vi "Image Marked Areas.vi"(7 "Calling VI Ref":refnum<vi>) -> ()   [LabVIEW 2020]
uses:
  <vilib>/Utility/miscctls.llb/LVPointTypeDef.ctl
  IMA Type Defs/IMA Actions.ctl
  Orca Flash Capture Manager/Orca Flash Capture Manager Controls/Orca Flash Capture Notifier Type.ctl
  Orca Flash Capture Manager/Orca Flash Capture Manager Controls/Orca Flash Capture Actions.ctl
  Orca Flash Capture Manager/Orca Flash Capture Manager Controls/Orca Flash Capture Switch Line Scan Modes.ctl
  Hardware Configuration/Hardware Configuration Controls/Device Function.ctl
  Hardware Configuration/Hardware Configuration Controls/Device Type.ctl
  IMA Type Defs/IMA Marked Positions.ctl
  Wide Field Drift Correction/WFDC Controls/WFDC Notifier Element.ctl
  Wide Field Drift Correction/WFDC Controls/WFDC Actions.ctl
  <vilib>/vision/Image Controls.llb/IMAQ Image.ctl
  Wide Field Drift Correction/WFDC Controls/WFDC External Sync.ctl
  Wide Field Drift Correction/WFDC Controls/WFDC Cycle Pause.ctl
  Wide Field Drift Correction/WFDC Controls/WFDC Status.ctl
  Device Library/Stages/Stages Controls/Stage Actions.ctl
  <vilib>/Utility/error.llb/whitespace.ctl
  8d6d82c7-2c11-4586-8521-e073de89416a.vi
  Device Library/Microscopes/Polymorphic Microscope Messenger/Set Obj Z Pos.vi
  Device Library/Microscopes/Polymorphic Microscope Messenger/Get Obj Z Pos.vi
panel:
  in  "Acquisition Control":enum32{"Capture", "Capture All", "Abort"}(radio)
  in  "Skip":bool
  in  "Clear All":bool
  in  "Clear Selected":bool
  in  "Mark Point":bool
  in  "Marked Positions":i32(listbox)
  in  "Quit":bool
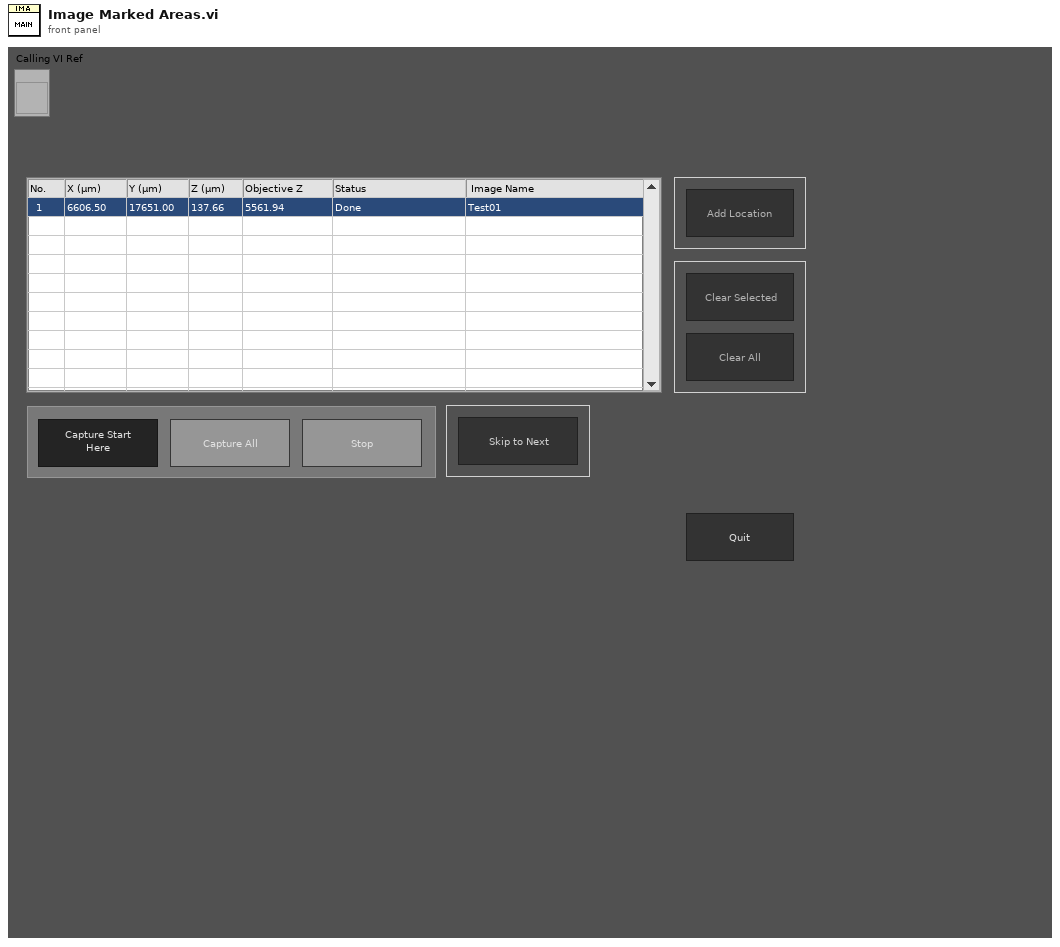
[diagram p1: front panel]
types:
  T1 = typedef "Orca Flash Capture Notifier Type.ctl" = cluster{"Actions":T2, "Running?":bool, "Preview Exposure (s)":dbl, "Capture Exposure (s)":dbl, "Cycles":u16, "Frames":u32, "No. of Z Steps":u16, "Z Step Size (µm)":dbl, "Base Path":path, "Init Z Position (µm)":dbl, "Lasers Lines":string[], "Save Path":path, "Line Scan?":bool, "Line Scan Mode":T3, "Collect Metadata?":bool, "channelCode":u8, "setupName":string, "Presaved Metadata":path}
  T2 = typedef "Orca Flash Capture Actions.ctl" = enum16{"Idle", "Live Preview", "Capture", "Check File Name", "Laser On", "Laser Off", "Open Shutters", "Close Shutters", "Set Exposure Time", "Start Acquisition", "Update SubFolder", "Write Metadata", "Setup", "Camera", "Switch", "Step", "Cycle", "External Cycle Sync", "Abort", "Quit"}
  T3 = typedef "Orca Flash Capture Switch Line Scan Modes.ctl" = enum32{"Automatic", "Use Presets", "Manual"}
  T4 = typedef "IMA Actions.ctl" = enum16{"Add Position", "Update Saved", "Remove Position", "Capture All", "Capture Here", "Move to Position", "Update Name", "Capture", "Switch", "Clear All", "Abort", "Exit Loop", "Quit"}
  T5 = enum16{"Always On", "Always Off", "Off While Running"}
  T6 = typedef "LVPointTypeDef.ctl" = cluster{"Horizontal":i16, "Vertical":i16}
  T7 = enum8{"Enabled", "Disabled", "Disabled and Grayed Out"}
  T8 = typedef "Device Function.ctl" = enum16{"Primary", "Secondary", "Overview", "Wide Field Drift Correction", "642 nm Excitation", "560 nm Excitation", "940 nm Excitation", "546 nm Excitation", "488 nm Excitation", "405 nm Excitation", "Objective Drift Correction", "4Pi Objective Lock", "Objective XY", "Objective Z", "Sample XY", "Sample Coarse Z", "Sample Z", "4Pi Lower", "4Pi Upper", "Mojo", "Adj Cavity", "Line Scanning", "Alert"}
  T9 = typedef "Device Type.ctl" = enum16{"AOTF", "Camera", "Deformable Mirror", "Laser", "Microscope Base", "Shutter", "Stage", "Waveform", "FPGA", "Email", "Filter Wheel", "Spinning Disk"}
  T10 = typedef "WFDC External Sync.ctl" = cluster{"Cycle Sync":T11, "Z Offset":dbl, "WFDC Status":T12}
  T11 = typedef "WFDC Cycle Pause.ctl" = enum16{"Pause Requested", "Paused", "Resume Requested", "Resumed"}
  T12 = typedef "WFDC Status.ctl" = enum16{"Idle", "Busy", "DC Active", "Error", "Canceled"}
  T13 = typedef "WFDC Notifier Element.ctl" = cluster{"WFDC Actions":T14, "Initial XYZ Positions":dbl[], "Ref Images":T15[], "Calibration (slope, inter)":dbl[], "Base Path":path, "Latest Scan Path":path, "Error":errorcluster, "XYZ Drift":dbl[]}
  T14 = typedef "WFDC Actions.ctl" = enum16{"Error Check", "Remote Start", "Move to Pos", "Pre Start Get Drift", "Pre Start Check Drift", "Pre Start Z Drift", "Pre Start XY Drift", "Pre Start ReFocus", "Setup New DC", "Setup Camera", "Get Ref Images", "Calc Calibration", "Switch Tabs", "Get Drift", "Z Drift", "XY Drift", "Start Cycle", "Stop DC", "Abort Remote", "Exit Loop", "Set Error", "Generate Calibration", "Quit"}
  T15 = typedef "IMAQ Image.ctl" = refnum<image>
  T16 = typedef "IMA Marked Positions.ctl" = cluster{"XYZ Positions":string[][], "File Paths":string[]}
  T17 = enum32{"Invalid", "Standard", "Closed", "Hidden", "Minimized", "Maximized"}
  T18 = typedef "Stage Actions.ctl" = enum16{"Get Position", "MVR", "MOVE", "HALT", "ONTARGET", "ERROR", "REFERENCE", "INIT", "VELOCITY", "STATUS", "EXIT", "HOME", "ZEROPOS", "NANOPOS", "ANALOG", "QUIT"}
  T19 = typedef "whitespace.ctl" = u16
  T20 = typedef "LVRectTypeDef.ctl" = cluster{"Left":i16, "Top":i16, "Right":i16, "Bottom":i16}
  T21 = typedef "LVBoundsTypeDef.ctl" = cluster{"Width":u32, "Height":u32}
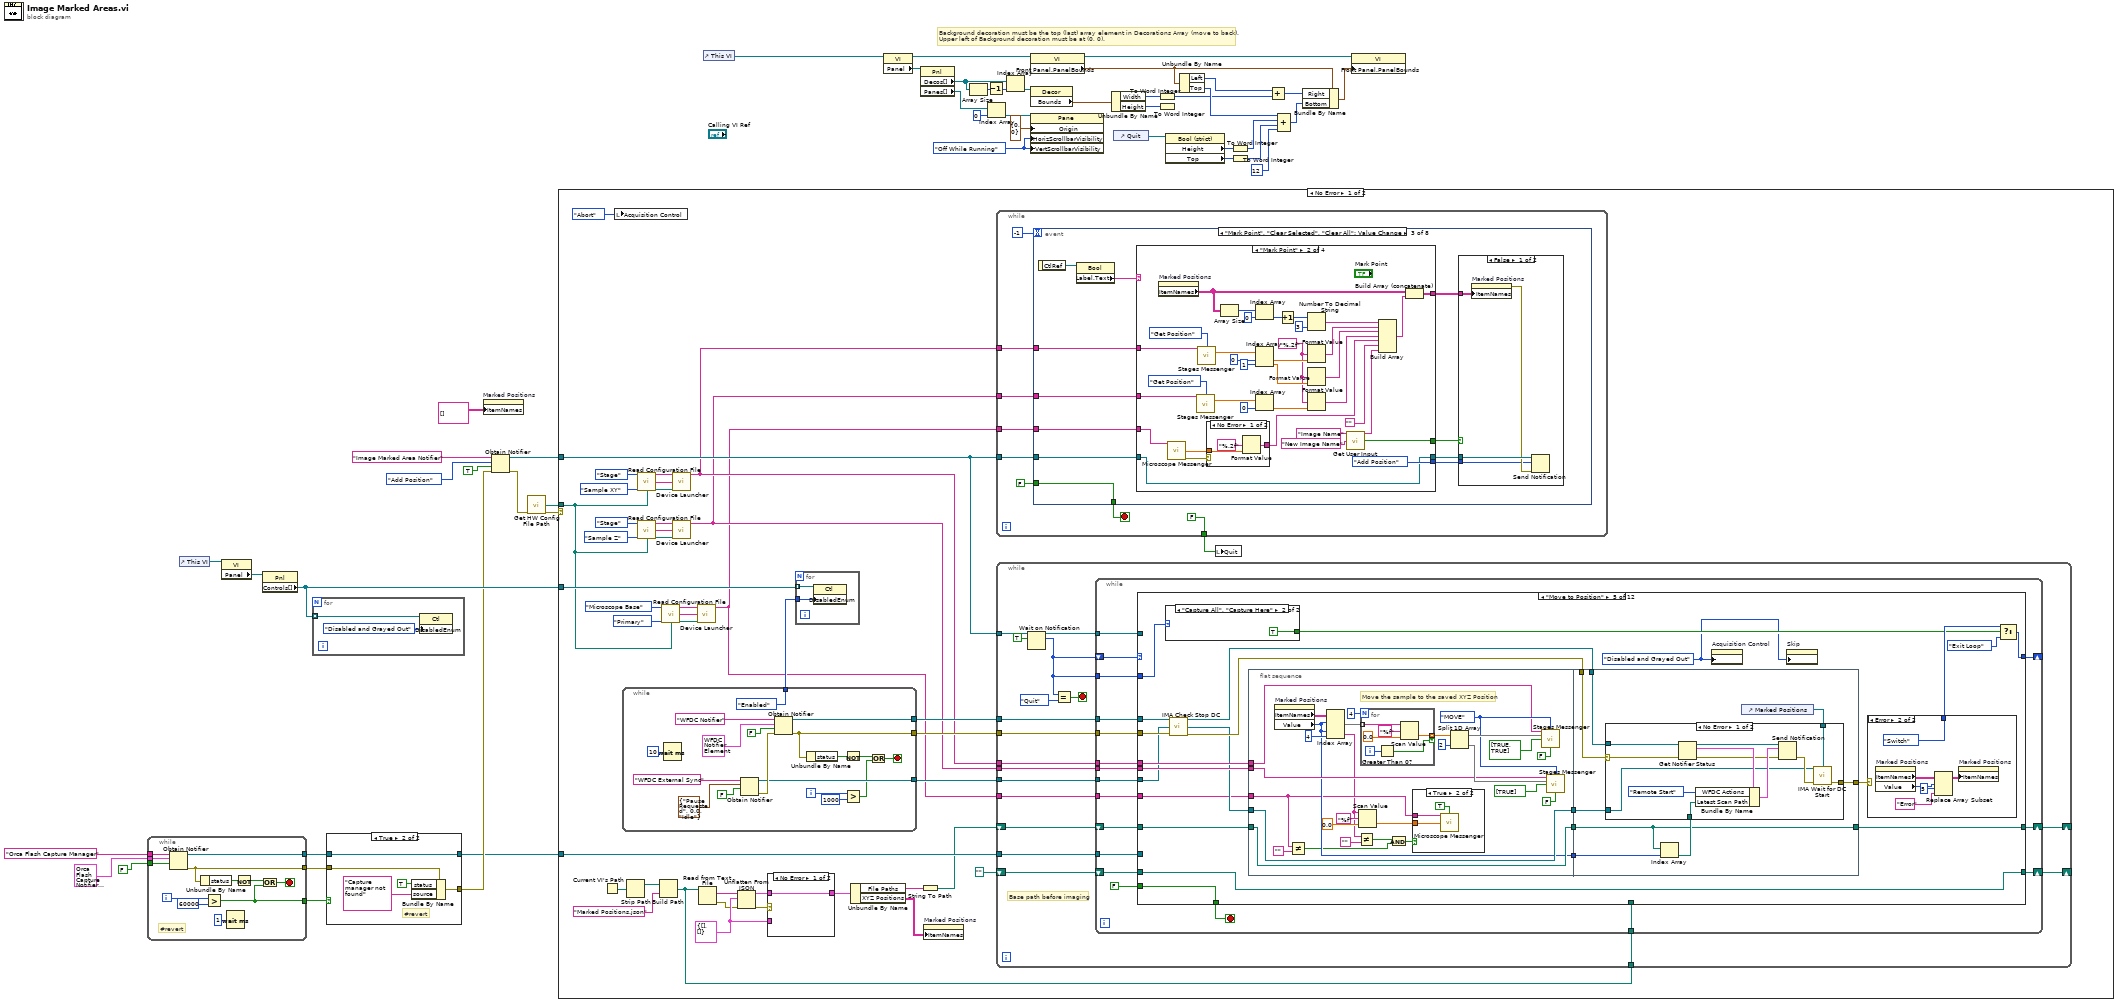
[diagram p0: block diagram]
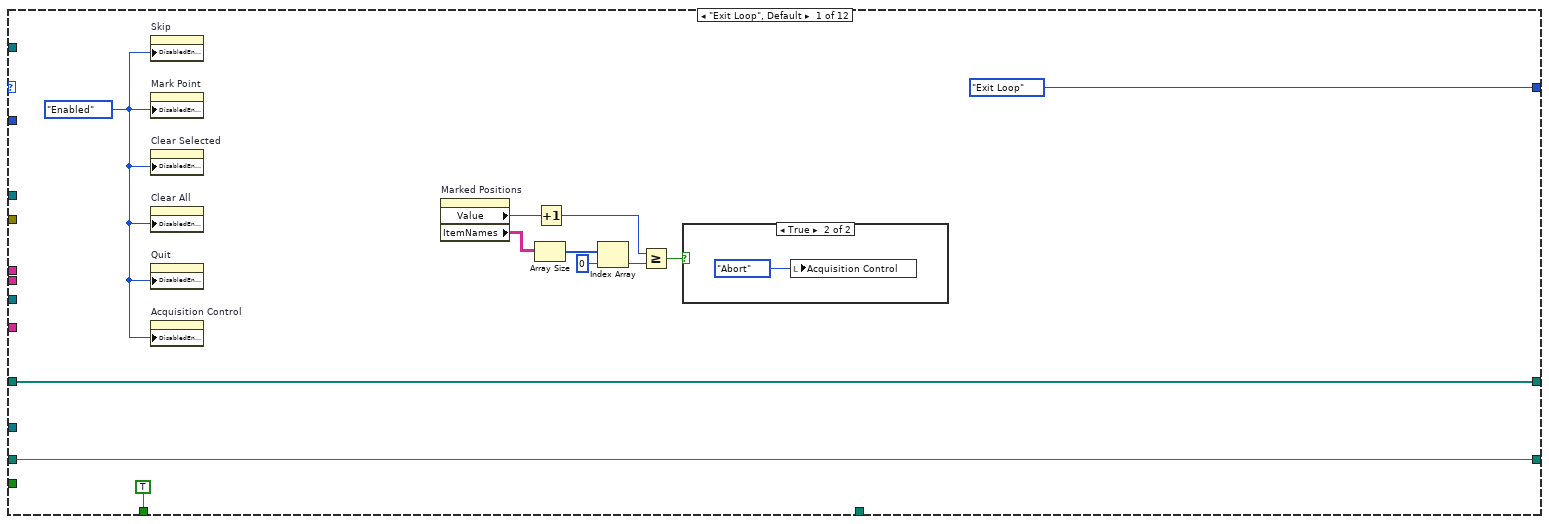
[diagram p4: hidden frame]
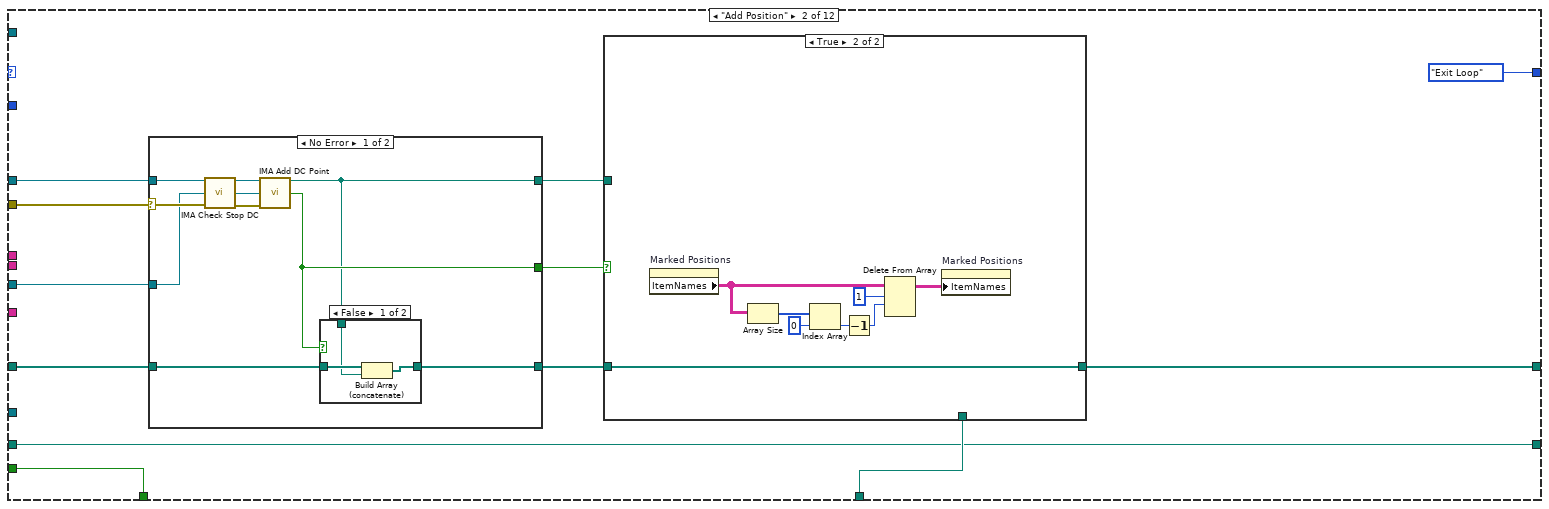
[diagram p6: hidden frame]
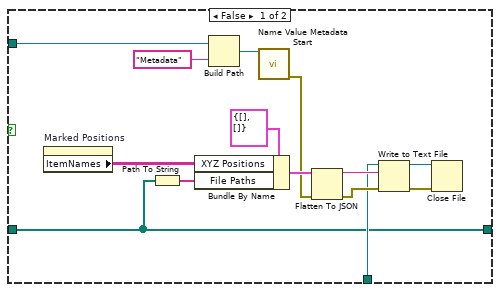
[diagram p7: hidden frame]
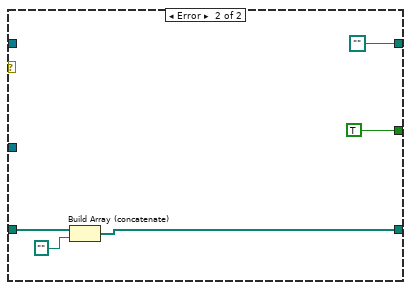
[diagram p9: hidden frame]
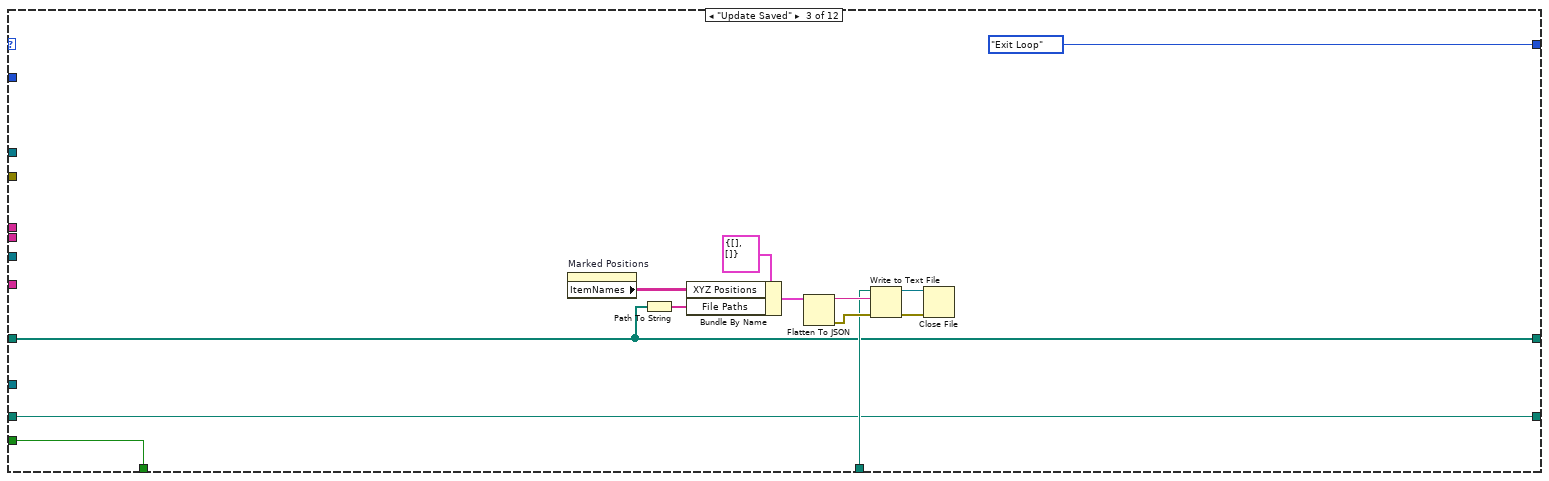
[diagram p10: hidden frame]
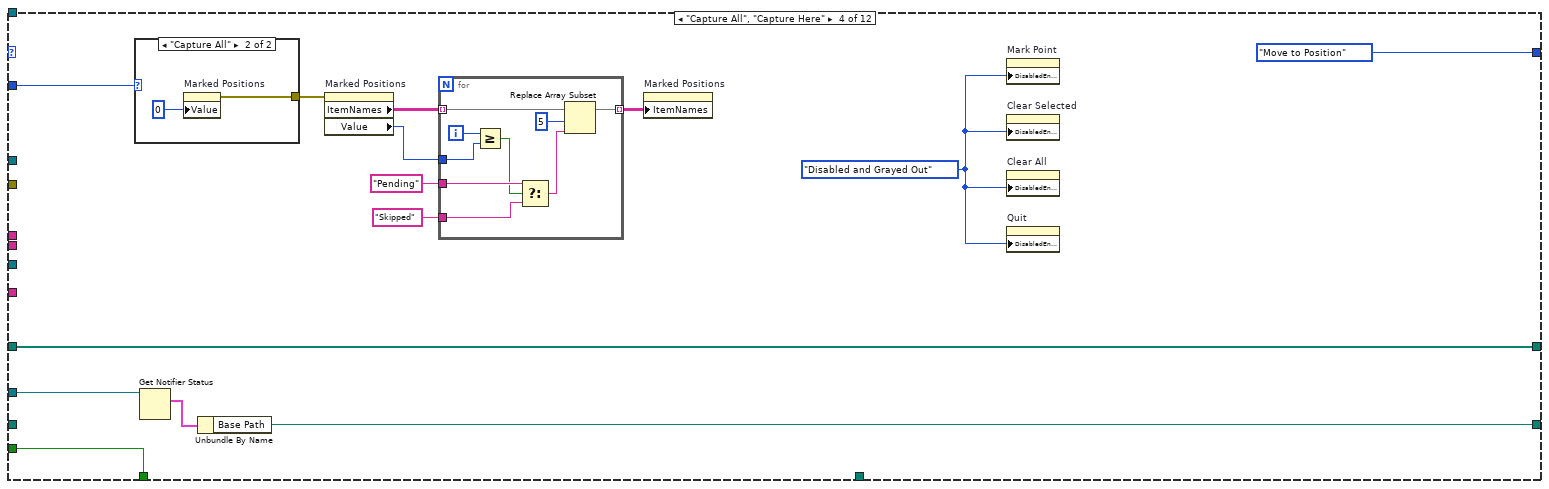
[diagram p11: hidden frame]
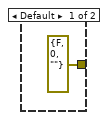
[diagram p12: hidden frame]
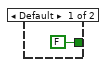
[diagram p13: hidden frame]
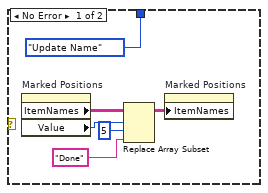
[diagram p14: hidden frame]
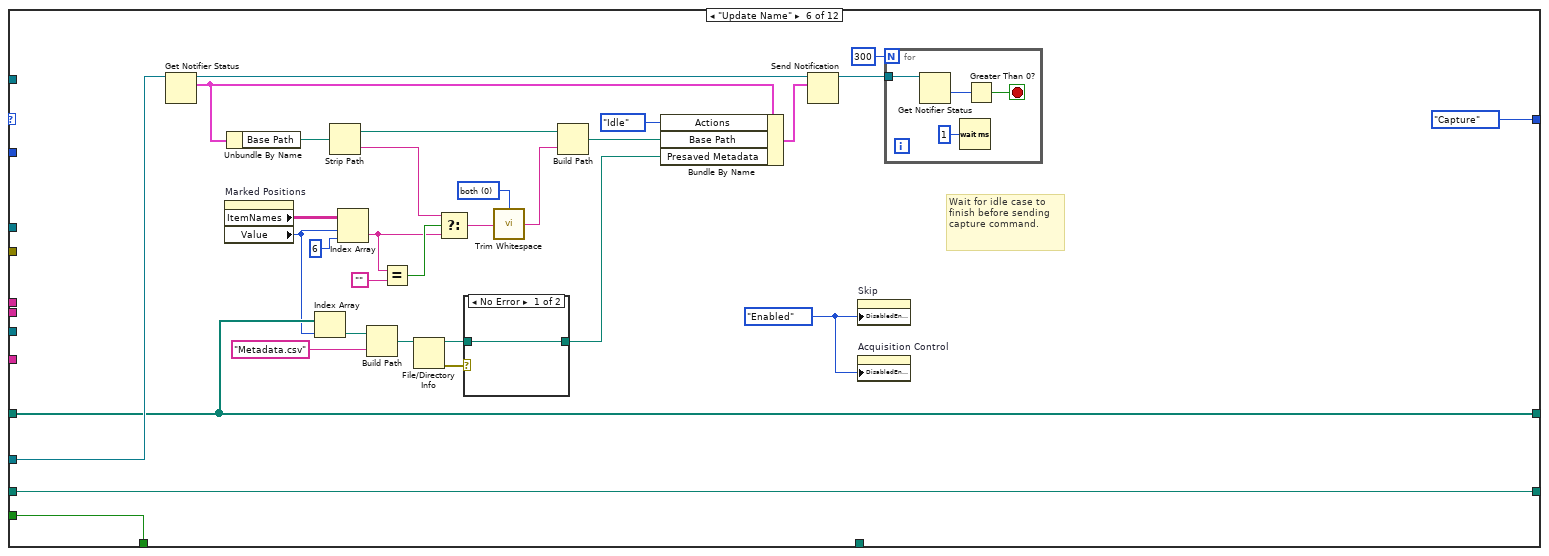
[diagram p17: hidden frame]
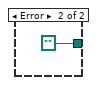
[diagram p18: hidden frame]
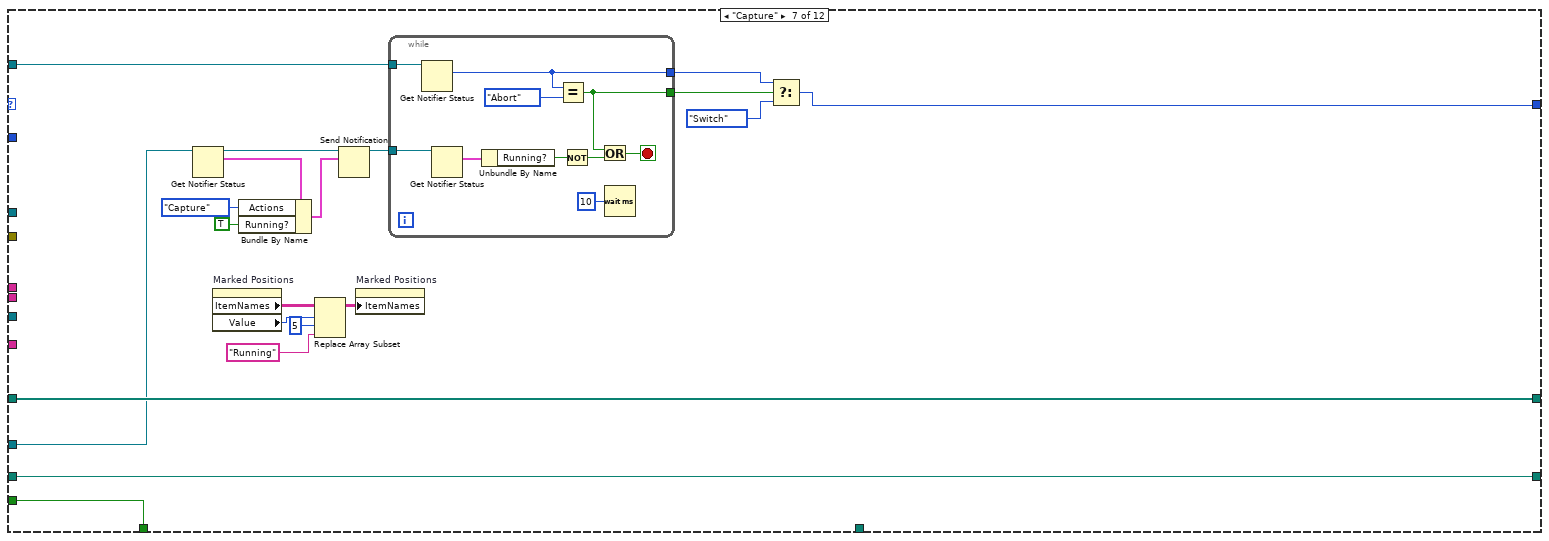
[diagram p19: hidden frame]
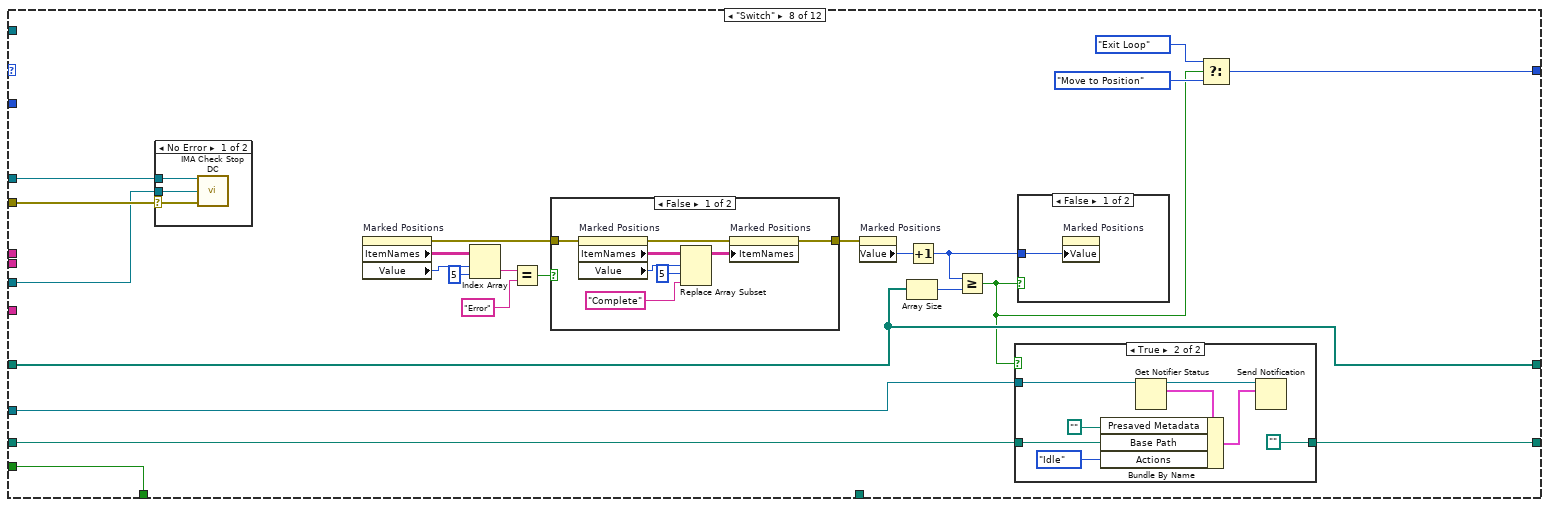
[diagram p20: hidden frame]
diagram:
  w29 = T5."Off While Running" ("Vertical Scrollbar Visibility")
  # "Background decoration must be the top (last) array element in Decorations Array (move to back).\nUpper left of Background decoration must be at (0, 0)."
  n1 = while {
    tunnel: FALSE ("create if not found? (T)") -> [w60]
    tunnel: "Orca Flash Capture Manager" ("name (unnamed)") -> [w59]
    tunnel: T1 {"Actions"=enum."Live Preview", "Running?"=FALSE, "Preview Exposure (s)"=0.1, "Capture Exposure (s)"=0.1, "Cycles"=1, "Frames"=0, "No. of Z Steps"=0, "Z Step Size (µm)"=0.0, "Base Path"=path "", "Init Z Position (µm)"=0.0, "Lasers Lines"=[], "Save Path"=path "", "Line Scan?"=FALSE, "Line Scan Mode"=enum."Automatic", "Collect Metadata?"=FALSE, "channelCode"=0, "setupName"="", "Presaved Metadata"=path ""} ("4Pi Capture Notifier Type") -> [w58]
    tunnel: [w54] -> w4
    tunnel: [w51] -> w5
    tunnel: [w49] -> w3
    i -> [w57]
    stop <- w50 stop-if-true
    # "#revert"
    n2 = Obtain Notifier(name (unnamed)=w59, notification data type=w58, create if not found? (T)=w60) -> (notifier out=w54:refnum<notifier>, error out=w49:errorcluster)  [unwired: 1 in, 1 out]
    n3 = Unbundle By Name(w49) -> ("status"=w53:bool)
    n4 = Greater?(x=w57, y=60000) -> (0:w51:bool)
    n5 = Wait (ms)(milliseconds to wait=u32 1) -> ()  [unwired: 1 out]
    n6 = Not(x=w53) -> (.not. x?=w52:bool)
    n7 = Or(x=w52, y=w51) -> (x .or. y?=w50:bool)
  }
  n8 = control-ref of="This VI"() -> (w11:refnum<vi>)
  n9 = property class="VI"(reference=w11) -> ("Panel"=w10:refnum<vi>)  [unwired: 1 in, 2 out]
  n10 = property class="Pnl"(reference=w10) -> ("Controls[]"=w9:refnum<vi>[])  [unwired: 1 in, 2 out]
  n11 = for {
    tunnel: w9 -> [w62] mode=indexing
    n12 = property class="Ctl"(reference=w62, "DisabledEnum"=T7."Disabled and Grayed Out" ("Disabled")) -> ()  [unwired: 1 in, 2 out]
  }
  n13 = case shown="True" w5 {
    tunnel: [w64 w67] -> w2
    tunnel: w4 -> [w63 w66]
    tunnel: [w63 w66] -> w1
    tunnel: w3 -> [w64 w65]
    frame False {
    }
    frame True {
      # "#revert"
      n14 = Bundle By Name(cluster=w65, "status"=TRUE, "source"="Capture manager not found") -> (w67:errorcluster)
    }
  }
  n15 = property on="Marked Positions" class="MCListbox (strict)"("ItemNames"=string[][] [] ("Item Names")) -> ()  [unwired: 2 in, 2 out]
  n16 = Obtain Notifier(name (unnamed)="Image Marked Area Notifier", notification data type=IMA_Actions."Add Position" ("Actions"), create if not found? (T)=TRUE, error in (no error)=w2) -> (notifier out=w13:refnum<notifier>, error out=w14:errorcluster)  [unwired: 1 out]
  n17 = call "Get HW Config File Path.vi"("Error"=w14) -> ("File Path"=w47:path, "Error"=w48:errorcluster)  [unwired: 13 in]
  n18 = case shown="No Error" w48 {
    selector: w48 -> [_ w703]
    tunnel: w47 -> [w71 _]
    tunnel: w13 -> [w100 w704]
    tunnel: w9 -> [w94 _]
    tunnel: w1 -> [w92 _]
    frame No Error {
      w88 = T16 {"XYZ Positions"=[], "File Paths"=[]} ("Marked Positions")
      n19 = Current VI's Path() -> (path=w87:path)
      n20 = local write "Acquisition Control"(enum32{"Capture", "Capture All", "Abort"}."Abort" ("Acquisition Control")) -> ()
      n21 = while {
        tunnel: [w130] -> w99
        tunnel: [w118] -> w98
        tunnel: [w125] -> w97
        tunnel: [T7."Enabled" ("Disabled")] -> w93
        i -> [w123]
        stop <- w117 stop-if-true
        n22 = Wait (ms)(milliseconds to wait=u32 10) -> ()  [unwired: 1 out]
        n23 = Obtain Notifier(name (unnamed)="WFDC External Sync", notification data type=T10 {"Cycle Sync"=enum."Pause Requested", "Z Offset"=0.0, "WFDC Status"=enum."Idle"} ("WFDC External Sync"), create if not found? (T)=FALSE) -> (notifier out=w125:refnum<notifier>, error out=w126:errorcluster)  [unwired: 1 in, 1 out]
        n24 = Obtain Notifier(name (unnamed)="WFDC Notifier", notification data type=T13 {"WFDC Actions"=enum."Error Check", "Initial XYZ Positions"=[], "Ref Images"=[], "Calibration (slope, inter)"=[], "Base Path"=path "", "Latest Scan Path"=path "", "Error"={"status"=FALSE, "code"=0, "source"=""}, "XYZ Drift"=[]} ("WFDC Notifier Element"), create if not found? (T)=FALSE, error in (no error)=w126) -> (notifier out=w130:refnum<notifier>, error out=w118:errorcluster)  [unwired: 1 out]
        n25 = Unbundle By Name(w118) -> ("status"=w121:bool)
        n26 = Not(x=w121) -> (.not. x?=w120:bool)
        n27 = Greater?(x=w123, y=1000) -> (0:w119:bool)
        n28 = Or(x=w120, y=w119) -> (x .or. y?=w117:bool)
      }
      n29 = Strip Path(path=w87) -> (stripped path=w81:path)  [unwired: 1 out]
      n30 = call "Read Configuration File.vi"("Device Type"=Device_Type."Stage", "Device Function"=Device_Function."Sample XY", "Config File Path"=w71) -> ("Unique Notifier Name"=w109:string, "Device Ports/IDs/Channels"=w111:string[], "Device Engine Path"=w110:path)  [unwired: 9 in, 1 out]
      n31 = call "Read Configuration File.vi"("Device Type"=Device_Type."Stage", "Device Function"=Device_Function."Sample Z", "Config File Path"=w71) -> ("Unique Notifier Name"=w103:string, "Device Ports/IDs/Channels"=w101:string[], "Device Engine Path"=w102:path)  [unwired: 9 in, 1 out]
      n32 = Build Path(base path=w81, name or relative path="Marked Positions.json") -> (appended path=w79:path)
      n33 = call "Read Configuration File.vi"("Device Type"=Device_Type."Microscope Base", "Device Function"=Device_Function."Primary", "Config File Path"=w71) -> ("Unique Notifier Name"=w74:string, "Device Ports/IDs/Channels"=w76:string[], "Device Engine Path"=w75:path)  [unwired: 9 in, 1 out]
      n34 = call "Device Launcher.vi"("Notifier Name"=w109, "Device Ports/IDs/Channels"=w111, "Device Engine Path"=w110) -> ("Notifier Name"=w96:string)  [unwired: 11 in, 1 out]
      n35 = call "Device Launcher.vi"("Notifier Name"=w103, "Device Ports/IDs/Channels"=w101, "Device Engine Path"=w102) -> ("Notifier Name"=w95:string)  [unwired: 11 in, 1 out]
      n36 = call "Device Launcher.vi"("Notifier Name"=w74, "Device Ports/IDs/Channels"=w76, "Device Engine Path"=w75) -> ("Notifier Name"=w70:string)  [unwired: 11 in, 1 out]
      n37 = Read from Text File(file (use dialog)=w79) -> (text=w83:string, error out=w84:errorcluster)  [unwired: 3 in, 2 out]
      n38 = Unflatten From JSON(JSON string=w83, type and defaults=w88, error in (no error)=w84) -> (value=w86:T16, error out=w85:errorcluster)  [unwired: 4 in]
      n39 = case shown="No Error" w85 {
        tunnel: w86 -> [w112 _]
        tunnel: [w112 w113] -> w89
        tunnel: w88 -> [_ w113]
        frame No Error {
        }
        frame Error {
        }
      }
      n40 = for {
        tunnel: w94 -> [w115] mode=indexing
        tunnel: w93 -> [w114]
        n41 = property class="Ctl"(reference=w115, "DisabledEnum"=w114) -> ()  [unwired: 1 in, 2 out]
      }
      n42 = Unbundle By Name(w89) -> ("File Paths"=w91:string[], "XYZ Positions"=w90:string[][])
      n43 = String To Path(string=w91) -> (path=w80:path[])
      n44 = property on="Marked Positions" class="MCListbox (strict)"("ItemNames"=w90) -> ()  [unwired: 2 in, 2 out]
      n45 = while {
        tunnel: [FALSE] -> w106
        tunnel: w96 -> [w555]
        tunnel: w95 -> [w554]
        tunnel: w100 -> [w553]
        tunnel: w70 -> [w552]
        stop <- w557 stop-if-true
        n46 = event shown="[2] \"Mark Point\", \"Clear Selected\", \"Clear All\": Value Change" {
          selector: _ -> [_ _ _ _ _ _ _ _]
          dyn-events: _ -> [_ _ _ _ _ _ _ _]
          timeout: -1 -> [_ _ _ _ _ _ _ _]
          tunnel: FALSE -> [w560 w564 w576 w654 w659 w664 w686 _]
          tunnel: [w560 w564 w576 w654 w659 w664 w686 w697] -> w557
          tunnel: w555 -> [_ _ w573 _ _ _ _ _]
          tunnel: w554 -> [_ _ w572 _ _ _ _ _]
          tunnel: w553 -> [_ _ w570 w653 w657 w662 w685 w696]
          tunnel: w552 -> [_ _ w566 _ _ _ _ _]
          event Timeout {
            n47 = event-data() -> ()  [unwired: 1 in, 1 out]
          }
          event Application Instance Close? {
            n48 = event-data() -> ()  [unwired: 1 in, 1 out]
            n49 = control-ref of="This VI"() -> (w561:refnum<vi>)
            n50 = invoke class="VI" method="FP.Open"(reference=w561, "Activate"=TRUE ("Activate?"), "State"=T17."Standard") -> ()  [unwired: 2 in, 5 out]
            n51 = event-data("Discard?"=TRUE) -> ()  [unwired: 1 in, 1 out]
          }
          event "Mark Point", "Clear Selected", "Clear All": Value Change {
            n52 = event-data() -> ("CtlRef"=w575:refnum<vi>)  [unwired: 1 in]
            n53 = property class="Bool"(reference=w575) -> ("Label.Text"=w571:string)  [unwired: 1 in, 2 out]
            n54 = case shown="\"Mark Point\"" w571 {
              tunnel: [w584 w605 w635 w644] -> w574
              tunnel: w573 -> [_ w603 _ _]
              tunnel: w572 -> [_ w600 _ _]
              tunnel: w570 -> [w583 w586 w632 w639]
              tunnel: [w583 w586 w630 w639] -> w569
              tunnel: [IMA_Actions."Exit Loop" ("notification") IMA_Actions."Add Position" ("notification") IMA_Actions."Exit Loop" ("notification") w638] -> w568
              tunnel: [FALSE ("Canceled?") w591 FALSE ("Canceled?") FALSE ("Canceled?")] -> w567
              tunnel: w566 -> [_ w589 _ _]
              frame Default {
                n55 = property on="Marked Positions" class="MCListbox (strict)"() -> ("ItemNames"=w584:string[][])  [unwired: 2 in, 2 out]
              }
              frame "Mark Point" {
                w602 = "%.2f" ("format string")
                n56 = property on="Marked Positions" class="MCListbox (strict)"() -> ("ItemNames"=w607:string[][])  [unwired: 2 in, 2 out]
                n57 = call-poly "Microscope Messenger.vi"("Notifier Name In"=w589) -> ("Obj Z Pos"=w587:dbl, "Error Out"=w588:errorcluster)  [unwired: 12 in, 1 out]
                n58 = call "Stages Messenger.vi"("Stage Notifier Name"=w600, "Actions"=Stage_Actions."Get Position") -> ("Positions"=w599:dbl[])  [unwired: 10 in, 3 out]
                n59 = call "Stages Messenger.vi"("Stage Notifier Name"=w603, "Actions"=Stage_Actions."Get Position") -> ("Positions"=w604:dbl[])  [unwired: 10 in, 3 out]
                n60 = case shown="No Error" w588 {
                  tunnel: w587 -> [w623 _]
                  tunnel: [w621 ""] -> w585
                  frame No Error {
                    n61 = Format Value(format string="%.2f", value (0)=w623) -> (output string=w621:string)  [unwired: 1 in]
                  }
                  frame Error {
                  }
                }
                n62 = Array Size(array=w607) -> (size(s)=w613:i32[])
                n63 = Index Array(array=w613, index=0) -> (element=w611:i32)
                n64 = Index Array(array=w604, index #1=0 ("index"), index #2=1 ("index")) -> (element #1=w617:dbl, element #2=w616:dbl)
                n65 = Index Array(array=w599, index=0) -> (element=w597:dbl)
                n66 = Increment(x=w611) -> (x+1=w615:i32)
                n67 = Number To Decimal String(number=w615, width (-)=i16 3) -> (decimal integer string=w610:string)
                n68 = Format Value(format string=w602, value (0)=w617) -> (output string=w608:string)  [unwired: 1 in]
                n69 = Format Value(format string=w602, value (0)=w616) -> (output string=w609:string)  [unwired: 1 in]
                n70 = Format Value(format string=w602, value (0)=w597) -> (output string=w596:string)  [unwired: 1 in]
                n71 = call "Get User Input.vi"("Window Title"="Image Name", "Dialog Message"="New Image Name") -> ("User Input"=w592:string, "Canceled?"=w591:bool)  [unwired: 11 in, 1 out]
                n72 = Build Array(w610, w608, w609, w596, w585, "", w592) -> (w606:string[])
                n73 = Build Array (concatenate)(w607, w606) -> (w605:string[][])
              }
              frame "Clear Selected" {
                n74 = Send Notification(notification=IMA_Actions."Remove Position", notifier=w632) -> (notifier out=w630:refnum<notifier>, error out=w627:errorcluster)  [unwired: 1 in]
                n75 = call "Stall Data Flow.vim"("value in"=w627, "milliseconds to wait"=u32 25) -> ("value out"=w626:errorcluster)  [unwired: 1 out]
                n76 = property on="Marked Positions" class="MCListbox (strict)"() -> ("ItemNames"=w636:string[][])  [unwired: 2 in, 2 out]
                n77 = property on="Marked Positions" class="MCListbox (strict)"(error in=w626) -> ("Value"=w633:i32)  [unwired: 1 in, 2 out]
                n78 = Delete From Array(array=w636, length=1, index (row)=w633) -> (array with subset deleted=w635:string[][])  [unwired: 1 in, 1 out]
              }
              frame "Clear All" {
                n79 = Two Button Dialog(message="Clear all marked positions?", 1:"Cancel" ("F button name (\"Cancel\")"), 2:"Okay" ("T button name (\"OK\")")) -> (T button?=w640:bool)
                n80 = case shown="True" w640 {
                  tunnel: [w646 string[][] []] -> w644
                  tunnel: [IMA_Actions."Exit Loop" ("notification") IMA_Actions."Clear All" ("notification")] -> w638
                  frame False {
                    n81 = property on="Marked Positions" class="MCListbox (strict)"() -> ("ItemNames"=w646:string[][])  [unwired: 2 in, 2 out]
                  }
                  frame True {
                  }
                }
              }
            }
            n82 = case shown="False" w567 {
              tunnel: w574 -> [w580 _]
              tunnel: w569 -> [w579 _]
              tunnel: w568 -> [w577 _]
              frame False {
                n83 = property on="Marked Positions" class="MCListbox (strict)"("ItemNames"=w580) -> (error out=w578:errorcluster)  [unwired: 2 in, 1 out]
                n84 = Send Notification(notification=w577, notifier=w579, error in (no error)=w578) -> ()  [unwired: 2 out]
              }
              frame True {
              }
            }
          }
          event "Marked Positions": Double Click {
            n85 = event-data() -> ()  [unwired: 1 in, 1 out]
            n86 = Two Button Dialog(message="Move to marked position?", 1:"Cancel" ("F button name (\"Cancel\")"), 2:"Yes" ("T button name (\"OK\")")) -> (T button?=w649:bool)
            n87 = case shown="True" w649 {
              tunnel: w653 -> [_ w656]
              frame False {
              }
              frame True {
                n88 = Send Notification(notification=IMA_Actions."Move to Position", notifier=w656) -> ()  [unwired: 1 in, 2 out]
              }
            }
          }
          event "Marked Positions": Edit Cell {
            n89 = event-data() -> ()  [unwired: 1 in, 6 out]
            n90 = Send Notification(notification=IMA_Actions."Update Saved", notifier=w657) -> ()  [unwired: 1 in, 2 out]
          }
          event "Acquisition Control": Value Change {
            n91 = event-data() -> ("NewVal"=w663:enum32{"Capture", "Capture All", "Abort"})  [unwired: 1 in]
            n92 = case shown="\"Abort\", Default" w663 {
              tunnel: [IMA_Actions."Capture Here" ("t") IMA_Actions."Capture All" ("t") IMA_Actions."Abort" ("t")] -> w660
              tunnel: w662 -> [w666 w669 w671]
              tunnel: [w665 w668 w671] -> w661
              frame "Capture" {
                n93 = call "IMA Check and Stop.vi"("IMA Note In"=w666) -> ("IMA Note Out"=w665:refnum<notifier>)  [unwired: 13 in, 1 out]
              }
              frame "Capture All" {
                n94 = call "IMA Check and Stop.vi"("IMA Note In"=w669) -> ("IMA Note Out"=w668:refnum<notifier>)  [unwired: 13 in, 1 out]
              }
              frame "Abort", Default {
              }
            }
            n95 = Send Notification(notification=w660, notifier=w661) -> ()  [unwired: 1 in, 2 out]
          }
          event "Skip": Value Change {
            n96 = event-data() -> ()  [unwired: 1 in, 1 out]
            n97 = property on="Marked Positions" class="MCListbox (strict)"() -> ("Value"=w681:i32, "ItemNames"=w680:string[][])  [unwired: 2 in, 2 out]
            n98 = Send Notification(notification=IMA_Actions."Abort", notifier=w685) -> (notifier out=w683:refnum<notifier>)  [unwired: 1 in, 1 out]
            n99 = Increment(x=w681) -> (x+1=w674:i32)
            n100 = Array Size(array=w680) -> (size(s)=w679:i32[])
            n101 = for {
              N: 600 -> [_]
              tunnel: w683 -> [w694]
              tunnel: [w691] -> w673
              stop <- w692 stop-if-true
              n102 = Wait (ms)(milliseconds to wait=u32 10) -> ()  [unwired: 1 out]
              n103 = Get Notifier Status(notifier=w694) -> (notifier out=w691:refnum<notifier>, # waiting=w693:i32)  [unwired: 1 in, 3 out]
              n104 = Greater Than 0?(x=w693) -> (x > 0?=w692:bool)
            }
            n105 = Index Array(array=w679, index=0) -> (element=w677:i32)
            n106 = Decrement(x=w677) -> (x-1=w676:i32)
            n107 = Greater?(x=w674, y=w676) -> (0:w675:bool)
            n108 = case shown="False" w675 {
              tunnel: w674 -> [w689 _]
              tunnel: w673 -> [w688 _]
              frame False {
                n109 = property on="Marked Positions" class="MCListbox (strict)"("Value"=w689) -> ()  [unwired: 2 in, 2 out]
                n110 = Send Notification(notification=IMA_Actions."Capture Here", notifier=w688) -> ()  [unwired: 1 in, 2 out]
              }
              frame True {
              }
            }
          }
          event "Quit": Value Change {
            n111 = event-data() -> ("NewVal"=w697:bool)  [unwired: 1 in]
            n112 = Send Notification(notification=IMA_Actions."Quit", notifier=w696) -> ()  [unwired: 1 in, 2 out]
          }
        }
      }
      n113 = while {
        tunnel: w100 -> [w151]
        tunnel: w99 -> [w145]
        tunnel: w98 -> [w144]
        tunnel: w97 -> [w146]
        shift-right: [w142] -> _
        shift-left: w80 -> [w143]
        tunnel: w96 -> [w140]
        tunnel: w95 -> [w139]
        tunnel: w92 -> [w138]
        tunnel: w79 -> [w137]
        shift-right: [w136] -> _
        shift-left: path "" -> [w135]
        tunnel: w70 -> [w134]
        stop <- w148 stop-if-true
        # "Base path before imaging"
        n114 = Wait on Notification(notifier=w151, ignore previous (F)=TRUE) -> (notifier out=w147:refnum<notifier>, notification=w141:T4)  [unwired: 2 in, 2 out]
        n115 = Equal?(x=w141, y=IMA_Actions."Quit") -> (x = y?=w148:bool)
        n116 = while {
          shift-right: [w165] -> _
          shift-left: w141 -> [w168]
          tunnel: w147 -> [w169]
          tunnel: w146 -> [w164]
          tunnel: w145 -> [w154]
          tunnel: w144 -> [w153]
          shift-right: [w162] -> w142
          shift-left: w143 -> [w163]
          tunnel: w141 -> [w161]
          tunnel: w140 -> [w160]
          tunnel: w139 -> [w159]
          tunnel: w138 -> [w158]
          tunnel: w137 -> [w157]
          shift-right: [w156] -> w136
          shift-left: w135 -> [w155]
          tunnel: w134 -> [w152]
          stop <- w166 stop-if-true
          n117 = case shown="\"Move to Position\"" w168 {
            tunnel: w169 -> [_ _ _ _ _ _ w408 _ _ _ _ w544]
            tunnel: w154 -> [_ w191 _ _ w284 _ _ w452 _ _ _ w547]
            tunnel: w153 -> [_ w192 _ _ w283 _ _ w451 _ _ _ w545]
            tunnel: [TRUE w194 w248 w262 w297 w400 w426 w459 w498 w516 w537 TRUE] -> w166
            tunnel: FALSE -> [_ w194 w248 w262 w297 w400 w426 w459 w498 w516 w537 _]
            tunnel: [IMA_Actions."Exit Loop" ("y") IMA_Actions."Exit Loop" ("y") IMA_Actions."Exit Loop" ("y") IMA_Actions."Move to Position" ("y") w287 IMA_Actions."Capture" ("y") w420 w453 IMA_Actions."Exit Loop" ("y") IMA_Actions."Exit Loop" ("y") IMA_Actions."Exit Loop" ("y") IMA_Actions."Quit" ("y")] -> w165
            tunnel: w164 -> [_ w190 _ _ w280 _ _ w450 _ _ _ w546]
            tunnel: w163 -> [w180 w189 w237 w261 w295 w380 w425 w441 w495 _ w536 w543]
            tunnel: [w180 w185 w237 w261 w294 w380 w425 w441 w487 w518 w536 w543] -> w162
            tunnel: w161 -> [_ _ _ w256 w278 _ _ _ _ _ _ _]
            tunnel: w160 -> [_ _ _ _ w291 _ _ _ _ _ _ _]
            tunnel: w159 -> [_ _ _ _ w292 _ _ _ _ _ _ _]
            tunnel: w158 -> [_ _ _ w258 _ w398 w419 w440 _ _ w533 _]
            tunnel: w157 -> [_ w187 w238 _ _ _ _ _ w483 w510 _ _]
            tunnel: [w178 w186 w236 w257 w285 w382 w413 w437 w482 w509 w535 w542] -> w156
            tunnel: w155 -> [w178 w186 w236 _ w285 w382 w413 w438 w482 w509 w535 w542]
            tunnel: w152 -> [_ _ _ _ w275 _ _ _ _ _ _ _]
            frame "Exit Loop", Default {
              w170 = T7."Enabled" ("Disabled")
              n118 = property on="Skip" class="Bool"("DisabledEnum"=w170) -> ()  [unwired: 2 in, 2 out]
              n119 = property on="Mark Point" class="Bool"("DisabledEnum"=w170) -> ()  [unwired: 2 in, 2 out]
              n120 = property on="Clear Selected" class="Bool"("DisabledEnum"=w170) -> ()  [unwired: 2 in, 2 out]
              n121 = property on="Clear All" class="Bool"("DisabledEnum"=w170) -> ()  [unwired: 2 in, 2 out]
              n122 = property on="Quit" class="Bool (strict)"("DisabledEnum"=w170) -> ()  [unwired: 2 in, 2 out]
              n123 = property on="Acquisition Control" class="RadioBtnsControl (strict)"("DisabledEnum"=w170) -> ()  [unwired: 2 in, 2 out]
              n124 = property on="Marked Positions" class="MCListbox (strict)"() -> ("Value"=w177:i32, "ItemNames"=w175:string[][])  [unwired: 2 in, 2 out]
              n125 = Array Size(array=w175) -> (size(s)=w173:i32[])
              n126 = Increment(x=w177) -> (x+1=w176:i32)
              n127 = Index Array(array=w173, index=0) -> (element=w171:i32)
              n128 = Greater Or Equal?(x=w176, y=w171) -> (x >= y?=w174:bool)
              n129 = case shown="True" w174 {
                frame False {
                }
                frame True {
                  n130 = local write "Acquisition Control"(enum32{"Capture", "Capture All", "Abort"}."Abort" ("Acquisition Control")) -> ()
                }
              }
            }
            frame "Add Position" {
              n131 = case shown="No Error" w192 {
                selector: w192 -> [w222 _]
                tunnel: w191 -> [w224 _]
                tunnel: w190 -> [w221 _]
                tunnel: w189 -> [w226 w235]
                tunnel: [w225 w234] -> w188
                tunnel: [w218 TRUE ("Canceled")] -> w184
                tunnel: [w217 path ""] -> w183
                frame No Error {
                  n132 = call "IMA Check Stop DC.vi"("WFDC Notifier"=w224, "WFDC External Sync"=w221, "Error"=w222) -> ("WFDC Notifier (Dup)"=w223:refnum<notifier>, "WFDC External Sync (Dup)"=w219:refnum<notifier>, "Error Out"=w220:errorcluster)  [unwired: 10 in]
                  n133 = call "IMA Add DC Point.vi"("WFDC Notifier"=w223, "WFDC External Sync"=w219, "Error"=w220) -> ("Scan Path"=w217:path, "Canceled"=w218:bool)  [unwired: 10 in, 1 out]
                  n134 = case shown="False" w218 {
                    tunnel: w226 -> [w229 w230]
                    tunnel: [w228 w230] -> w225
                    tunnel: w217 -> [w227 _]
                    frame False {
                      n135 = Build Array (concatenate)(w229, w227) -> (w228:path[])
                    }
                    frame True {
                    }
                  }
                }
                frame Error {
                  n136 = Build Array (concatenate)(w235, path "") -> (w234:path[])
                }
              }
              n137 = case shown="True" w184 {
                tunnel: w188 -> [w199 w216]
                tunnel: w187 -> [w200 _]
                tunnel: [w199 w216] -> w185
                tunnel: w183 -> [w198 _]
                frame False {
                  n138 = property on="Marked Positions" class="MCListbox (strict)"() -> ("ItemNames"=w207:string[][])  [unwired: 2 in, 2 out]
                  n139 = Path To String(path=w199) -> (string=w206:string[])
                  n140 = Bundle By Name(cluster=T16 {"XYZ Positions"=[], "File Paths"=[]} ("Marked Positions"), "XYZ Positions"=w207, "File Paths"=w206) -> (w205:T16)
                  n141 = Build Path(base path=w198, name or relative path="Metadata") -> (appended path=w196:path)
                  n142 = call "Name Value Metadata Start.vi"("Metadata Save Path"=w196) -> ("Error Out"=w195:errorcluster)  [unwired: 14 in]
                  n143 = Flatten To JSON(anything=w205, error in (no error)=w195) -> (JSON string=w204:string, 11:w202:errorcluster)  [unwired: 1 in]
                  n144 = Write to Text File(file (use dialog)=w200, text=w204, error in=w202) -> (refnum out=w203:refnum<file>, error out=w201:errorcluster)  [unwired: 1 in, 1 out]
                  n145 = Close File(refnum=w203, error in=w201) -> ()  [unwired: 2 out]
                }
                frame True {
                  n146 = property on="Marked Positions" class="MCListbox (strict)"() -> ("ItemNames"=w214:string[][])  [unwired: 2 in, 2 out]
                  n147 = Array Size(array=w214) -> (size(s)=w213:i32[])
                  n148 = Index Array(array=w213, index=0) -> (element=w211:i32)
                  n149 = Decrement(x=w211) -> (x-1=w209:i32)
                  n150 = Delete From Array(array=w214, length=1, index (row)=w209) -> (array with subset deleted=w210:string[][])  [unwired: 1 in, 1 out]
                  n151 = property on="Marked Positions" class="MCListbox (strict)"("ItemNames"=w210) -> ()  [unwired: 2 in, 2 out]
                }
              }
            }
            frame "Update Saved" {
              n152 = property on="Marked Positions" class="MCListbox (strict)"() -> ("ItemNames"=w245:string[][])  [unwired: 2 in, 2 out]
              n153 = Path To String(path=w237) -> (string=w244:string[])
              n154 = Bundle By Name(cluster=T16 {"XYZ Positions"=[], "File Paths"=[]} ("Marked Positions"), "XYZ Positions"=w245, "File Paths"=w244) -> (w243:T16)
              n155 = Flatten To JSON(anything=w243) -> (JSON string=w242:string, 11:w240:errorcluster)  [unwired: 2 in]
              n156 = Write to Text File(file (use dialog)=w238, text=w242, error in=w240) -> (refnum out=w241:refnum<file>, error out=w239:errorcluster)  [unwired: 1 in, 1 out]
              n157 = Close File(refnum=w241, error in=w239) -> ()  [unwired: 2 out]
            }
            frame "Capture All", "Capture Here" {
              w249 = T7."Disabled and Grayed Out" ("Disabled")
              n158 = case shown="\"Capture All\"" w256 {
                tunnel: [errorcluster {"status"=FALSE, "code"=0, "source"=""} ("error out") w273] -> w255
                frame Default {
                }
                frame "Capture All" {
                  n159 = property on="Marked Positions" class="MCListbox (strict)"("Value"=0 ("Focus Row")) -> (error out=w273:errorcluster)  [unwired: 2 in, 1 out]
                }
              }
              n160 = Get Notifier Status(notifier=w258) -> (current notification=w259:T1)  [unwired: 1 in, 4 out]
              n161 = Unbundle By Name(w259) -> ("Base Path"=w257:path)
              n162 = property on="Marked Positions" class="MCListbox (strict)"(error in=w255) -> ("ItemNames"=w254:string[][], "Value"=w252:i32)  [unwired: 1 in, 2 out]
              n163 = for {
                tunnel: w254 -> [w271] mode=indexing
                tunnel: [w269] -> w253 mode=indexing
                tunnel: w252 -> [w267]
                tunnel: "Pending" -> [w266]
                tunnel: "Skipped" -> [w265]
                i -> [w268]
                n164 = Greater Or Equal?(x=w268, y=w267) -> (x >= y?=w264:bool)
                n165 = Select(t=w266, s=w264, f=w265) -> (s? t:f=w263:string)
                n166 = Replace Array Subset(array=w271, new element=w263, index=5) -> (w269:string[])
              }
              n167 = property on="Marked Positions" class="MCListbox (strict)"("ItemNames"=w253) -> ()  [unwired: 2 in, 2 out]
              n168 = property on="Mark Point" class="Bool"("DisabledEnum"=w249) -> ()  [unwired: 2 in, 2 out]
              n169 = property on="Clear Selected" class="Bool"("DisabledEnum"=w249) -> ()  [unwired: 2 in, 2 out]
              n170 = property on="Clear All" class="Bool"("DisabledEnum"=w249) -> ()  [unwired: 2 in, 2 out]
              n171 = property on="Quit" class="Bool (strict)"("DisabledEnum"=w249) -> ()  [unwired: 2 in, 2 out]
            }
            frame "Move to Position" {
              w276 = T7."Disabled and Grayed Out" ("Disabled")
              n172 = case shown="\"Capture All\", \"Capture Here\"" w278 {
                tunnel: [FALSE TRUE] -> w277
                frame Default {
                }
                frame "Capture All", "Capture Here" {
                }
              }
              n173 = call "IMA Check Stop DC.vi"("WFDC Notifier"=w284, "WFDC External Sync"=w280, "Error"=w283) -> ("WFDC Notifier (Dup)"=w281:refnum<notifier>, "WFDC External Sync (Dup)"=w279:refnum<notifier>, "Error Out"=w282:errorcluster)  [unwired: 10 in]
              n174 = flat-sequence {
                tunnel: [w325] -> w296
                tunnel: w295 -> [w325]
                tunnel: [w321] -> w293
                tunnel: w279 -> [w321]
                tunnel: w292 -> [w327]
                tunnel: w291 -> [w328]
                tunnel: [w319] -> w289
                tunnel: w275 -> [w318]
                tunnel: w296 -> [w355]
                tunnel: [w355] -> w294
                tunnel: w293 -> [w354]
                tunnel: w282 -> [w353]
                tunnel: w281 -> [w352]
                tunnel: w289 -> [w351]
                tunnel: [w350] -> w288
                frame #0 {
                  w329 = Stage_Actions."MOVE" ("Actions")
                  # "Move the sample to the saved XYZ Position"
                  n175 = property on="Marked Positions" class="MCListbox (strict)"() -> ("ItemNames"=w337:string[][], "Value"=w319:i32)  [unwired: 2 in, 2 out]
                  n176 = Not Equal?(x=w318, y="") -> (x != y?=w316:bool)
                  n177 = Index Array(array=w337, index (row) #1=w319, index (row) #2=w319, index (col) #2=4 ("disabled index (col)")) -> (element #1=w334:string[], element #2=w312:string)  [unwired: 1 in]
                  n178 = Not Equal?(x=w312, y="") -> (x != y?=w313:bool)
                  n179 = Scan Value(string=w312, format string="%f", default (0 dbl)=0.0) -> (value=w320:dbl)  [unwired: 1 out]
                  n180 = for {
                    N: 4 -> [_]
                    tunnel: w334 -> [w346] mode=indexing
                    tunnel: [w345] -> w333 mode=indexing if=w343
                    i -> [w344]
                    n181 = Greater Than 0?(x=w344) -> (x > 0?=w343:bool)
                    n182 = Scan Value(string=w346, format string="%f", default (0 dbl)=0.0) -> (value=w345:dbl)  [unwired: 1 out]
                  }
                  n183 = And(x=w313, y=w316) -> (x .and. y?=w315:bool)
                  n184 = case shown="True" w315 {
                    tunnel: w320 -> [_ w341]
                    tunnel: w318 -> [_ w340]
                    frame False {
                    }
                    frame True {
                      n185 = call-poly "Microscope Messenger.vi"("Notifier Name In"=w340, "Wait to Finish"=TRUE, "Obj Z Pos (um)"=w341) -> ()  [unwired: 11 in, 2 out]
                    }
                  }
                  n186 = Split 1D Array(array=w333, index=2) -> (first subarray=w331:dbl[], second subarray=w330:dbl[])
                  n187 = call "Stages Messenger.vi"("Stage Notifier Name"=w328, "Actions"=w329, "Setpoint"=w331, "Axis"=bool[] [TRUE, TRUE], "Exit While Busy?"=FALSE ("Wait for On Target? (F)")) -> ()  [unwired: 7 in, 4 out]
                  n188 = call "Stages Messenger.vi"("Stage Notifier Name"=w327, "Actions"=w329, "Setpoint"=w330, "Axis"=bool[] [TRUE], "Exit While Busy?"=FALSE ("Wait for On Target? (F)")) -> ()  [unwired: 7 in, 4 out]
                }
                frame #1 {
                  n189 = Index Array(array=w355, index=w351) -> (element=w356:path)
                  n190 = control-ref of="Marked Positions"() -> (w349:refnum<vi>)
                  n191 = case shown="No Error" w353 {
                    selector: w353 -> [w358 w369]
                    tunnel: w352 -> [w359 _]
                    tunnel: w354 -> [w357 _]
                    tunnel: w356 -> [w364 _]
                    tunnel: [w361 w369] -> w350
                    tunnel: w349 -> [w360 _]
                    frame No Error {
                      n192 = Get Notifier Status(notifier=w359, error in (no error)=w358) -> (notifier out=w368:refnum<notifier>, current notification=w367:T13, error out=w365:errorcluster)  [unwired: 2 out]
                      n193 = Bundle By Name(cluster=w367, "WFDC Actions"=WFDC_Actions."Remote Start", "Latest Scan Path"=w364) -> (w366:T13)
                      n194 = Send Notification(notification=w366, notifier=w368, error in (no error)=w365) -> (error out=w362:errorcluster)  [unwired: 1 out]
                      n195 = call "IMA Wait for DC Start.vi"("WFDC External Sync"=w357, "Marked Positions Ref"=w360, "Error"=w362) -> ("Error Out"=w361:errorcluster)  [unwired: 11 in, 1 out]
                    }
                    frame Error {
                    }
                  }
                }
              }
              n196 = property on="Acquisition Control" class="RadioBtnsControl (strict)"("DisabledEnum"=w276) -> ()  [unwired: 2 in, 2 out]
              n197 = property on="Skip" class="Bool"("DisabledEnum"=w276) -> ()  [unwired: 2 in, 2 out]
              n198 = case shown="Error" w288 {
                tunnel: [IMA_Actions."Update Name" ("t") IMA_Actions."Switch" ("y")] -> w286
                frame No Error {
                  n199 = property on="Marked Positions" class="MCListbox (strict)"() -> ("ItemNames"=w302:string[][], "Value"=w303:i32)  [unwired: 2 in, 2 out]
                  n200 = Replace Array Subset(array=w302, new element="Done" ("new element/subarray"), index (row)=w303, index (col)=5 ("disabled index (col)")) -> (w304:string[][])
                  n201 = property on="Marked Positions" class="MCListbox (strict)"("ItemNames"=w304) -> ()  [unwired: 2 in, 2 out]
                }
                frame Error {
                  n202 = property on="Marked Positions" class="MCListbox (strict)"() -> ("ItemNames"=w307:string[][], "Value"=w308:i32)  [unwired: 2 in, 2 out]
                  n203 = Replace Array Subset(array=w307, new element="Error" ("new element/subarray"), index (row)=w308, index (col)=5 ("disabled index (col)")) -> (w311:string[][])
                  n204 = property on="Marked Positions" class="MCListbox (strict)"("ItemNames"=w311) -> ()  [unwired: 2 in, 2 out]
                }
              }
              n205 = Select(t=w286, s=w277, f=IMA_Actions."Exit Loop" ("y")) -> (s? t:f=w287:T4)
            }
            frame "Update Name" {
              w370 = T7."Enabled" ("Disabled")
              w395 = T19 0 items=["both", "start of string", "end of string"] ("location (both)")
              # "Wait for idle case to finish before sending capture command."
              n206 = Get Notifier Status(notifier=w398) -> (notifier out=w397:refnum<notifier>, current notification=w392:T1)  [unwired: 1 in, 3 out]
              n207 = property on="Marked Positions" class="MCListbox (strict)"() -> ("ItemNames"=w393:string[][], "Value"=w379:i32)  [unwired: 2 in, 2 out]
              n208 = Unbundle By Name(w392) -> ("Base Path"=w396:path)
              n209 = Index Array(array=w380, index=w379) -> (element=w378:path)
              n210 = Strip Path(path=w396) -> (stripped path=w391:path, name=w385:string)
              n211 = Index Array(array=w393, index (row)=w379, index (col)=6 ("disabled index (col)")) -> (element=w384:string)
              n212 = Build Path(base path=w378, name or relative path="Metadata.csv") -> (appended path=w377:path)
              n213 = Equal?(x=w384, y="") -> (x = y?=w386:bool)
              n214 = File/Directory Info(path=w377) -> (path out=w375:path, error out=w376:errorcluster)  [unwired: 1 in, 5 out]
              n215 = Select(t=w385, s=w386, f=w384) -> (s? t:f=w383:string)
              n216 = case shown="No Error" w376 {
                tunnel: w375 -> [w405 _]
                tunnel: [w405 path ""] -> w374
                frame No Error {
                }
                frame Error {
                }
              }
              n217 = call <vilib>:"Trim Whitespace.vi"("string"=w383, "location (both)"=w395) -> ("trimmed string"=w390:string)
              n218 = Build Path(base path=w391, name or relative path=w390) -> (appended path=w389:path)
              n219 = Bundle By Name(cluster=w392, "Actions"=Orca_Flash_Capture_Actions."Idle", "Base Path"=w389, "Presaved Metadata"=w374) -> (w388:T1)
              n220 = Send Notification(notification=w388, notifier=w397) -> (notifier out=w372:refnum<notifier>)  [unwired: 1 in, 1 out]
              n221 = property on="Skip" class="Bool"("DisabledEnum"=w370) -> ()  [unwired: 2 in, 2 out]
              n222 = property on="Acquisition Control" class="RadioBtnsControl (strict)"("DisabledEnum"=w370) -> ()  [unwired: 2 in, 2 out]
              n223 = for {
                N: 300 -> [_]
                tunnel: w372 -> [w404]
                stop <- w402 stop-if-true
                n224 = Get Notifier Status(notifier=w404) -> (# waiting=w403:i32)  [unwired: 1 in, 4 out]
                n225 = Wait (ms)(milliseconds to wait=u32 1) -> ()  [unwired: 1 out]
                n226 = Greater Than 0?(x=w403) -> (x > 0?=w402:bool)
              }
            }
            frame "Capture" {
              n227 = Get Notifier Status(notifier=w419) -> (notifier out=w422:refnum<notifier>, current notification=w424:T1)  [unwired: 1 in, 3 out]
              n228 = property on="Marked Positions" class="MCListbox (strict)"() -> ("ItemNames"=w414:string[][], "Value"=w415:i32)  [unwired: 2 in, 2 out]
              n229 = Bundle By Name(cluster=w424, "Actions"=Orca_Flash_Capture_Actions."Capture", "Running?"=TRUE) -> (w421:T1)
              n230 = Replace Array Subset(array=w414, new element="Running" ("new element/subarray"), index (row)=w415, index (col)=5 ("disabled index (col)")) -> (w418:string[][])
              n231 = Send Notification(notification=w421, notifier=w422) -> (notifier out=w407:refnum<notifier>)  [unwired: 1 in, 1 out]
              n232 = property on="Marked Positions" class="MCListbox (strict)"("ItemNames"=w418) -> ()  [unwired: 2 in, 2 out]
              n233 = while {
                tunnel: w407 -> [w436]
                tunnel: w408 -> [w434]
                tunnel: [w431] -> w411
                tunnel: [w429] -> w410
                stop <- w432 stop-if-true
                n234 = Get Notifier Status(notifier=w434) -> (current notification=w429:T4)  [unwired: 1 in, 4 out]
                n235 = Get Notifier Status(notifier=w436) -> (current notification=w435:T1)  [unwired: 1 in, 4 out]
                n236 = Unbundle By Name(w435) -> ("Running?"=w433:bool)
                n237 = Equal?(x=w429, y=IMA_Actions."Abort") -> (x = y?=w431:bool)
                n238 = Not(x=w433) -> (.not. x?=w430:bool)
                n239 = Or(x=w431, y=w430) -> (x .or. y?=w432:bool)
                n240 = Wait (ms)(milliseconds to wait=u32 10) -> ()  [unwired: 1 out]
              }
              n241 = Select(t=w410, s=w411, f=IMA_Actions."Switch") -> (s? t:f=w420:T4)
            }
            frame "Switch" {
              n242 = case shown="No Error" w451 {
                selector: w451 -> [w479 _]
                tunnel: w452 -> [w480 _]
                tunnel: w450 -> [w478 _]
                frame No Error {
                  n243 = call "IMA Check Stop DC.vi"("WFDC Notifier"=w480, "WFDC External Sync"=w478, "Error"=w479) -> ()  [unwired: 10 in, 3 out]
                }
                frame Error {
                }
              }
              n244 = property on="Marked Positions" class="MCListbox (strict)"() -> (error out=w449:errorcluster, "ItemNames"=w443:string[][], "Value"=w444:i32)  [unwired: 2 in, 1 out]
              n245 = Index Array(array=w443, index (row)=w444, index (col)=5 ("disabled index (col)")) -> (element=w446:string)
              n246 = Equal?(x=w446, y="Error") -> (x = y?=w448:bool)
              n247 = case shown="False" w448 {
                tunnel: w449 -> [w471 w477]
                tunnel: [w469 w477] -> w442
                frame False {
                  n248 = property on="Marked Positions" class="MCListbox (strict)"(error in=w471) -> (error out=w470:errorcluster, "ItemNames"=w472:string[][], "Value"=w473:i32)  [unwired: 1 in, 1 out]
                  n249 = Replace Array Subset(array=w472, new element="Complete" ("new element/subarray"), index (row)=w473, index (col)=5 ("disabled index (col)")) -> (w476:string[][])
                  n250 = property on="Marked Positions" class="MCListbox (strict)"(error in=w470, "ItemNames"=w476) -> (error out=w469:errorcluster)  [unwired: 1 in, 1 out]
                }
                frame True {
                }
              }
              n251 = property on="Marked Positions" class="MCListbox (strict)"(error in=w442) -> ("Value"=w458:i32)  [unwired: 1 in, 2 out]
              n252 = Array Size(array=w441) -> (size(s)=w457:i32)
              n253 = Increment(x=w458) -> (x+1=w456:i32)
              n254 = Greater Or Equal?(x=w456, y=w457) -> (x >= y?=w439:bool)
              n255 = case shown="True" w439 {
                tunnel: w440 -> [_ w468]
                tunnel: w438 -> [w460 w465]
                tunnel: [w460 path ""] -> w437
                frame False {
                }
                frame True {
                  n256 = Get Notifier Status(notifier=w468) -> (notifier out=w467:refnum<notifier>, current notification=w466:T1)  [unwired: 1 in, 3 out]
                  n257 = Bundle By Name(cluster=w466, "Presaved Metadata"=path "", "Base Path"=w465, "Actions"=Orca_Flash_Capture_Actions."Idle") -> (w464:T1)
                  n258 = Send Notification(notification=w464, notifier=w467) -> ()  [unwired: 1 in, 2 out]
                }
              }
              n259 = case shown="False" w439 {
                tunnel: w456 -> [w481 _]
                frame False {
                  n260 = property on="Marked Positions" class="MCListbox (strict)"("Value"=w481) -> ()  [unwired: 2 in, 2 out]
                }
                frame True {
                }
              }
              n261 = Select(t=IMA_Actions."Exit Loop" ("y"), s=w439, f=IMA_Actions."Move to Position" ("y")) -> (s? t:f=w453:T4)
            }
            frame "Remove Position" {
              n262 = property on="Marked Positions" class="MCListbox (strict)"() -> ("Value"=w497:i32)  [unwired: 2 in, 2 out]
              n263 = property on="Marked Positions" class="MCListbox (strict)"() -> ("ItemNames"=w486:string[][])  [unwired: 2 in, 2 out]
              n264 = Delete From Array(array=w495, length=1, index=w497) -> (array with subset deleted=w487:path[])  [unwired: 1 out]
              n265 = Array Size(array=w486) -> (size(s)=w485:i32[])
              n266 = while {
                tunnel: w485 -> [w508]
                tunnel: [w500] -> w484
                i -> [w506]
                stop <- w502 stop-if-true
                n267 = property on="Marked Positions" class="MCListbox (strict)"() -> ("ItemNames"=w500:string[][])  [unwired: 2 in, 2 out]
                n268 = Wait (ms)(milliseconds to wait=u32 2) -> ()  [unwired: 1 out]
                n269 = Array Size(array=w500) -> (size(s)=w507:i32[])
                n270 = Greater?(x=w506, y=500) -> (0:w504:bool)
                n271 = Not Equal?(x=w507, y=w508) -> (x != y?=w503:bool)
                n272 = Or(x=w503, y=w504) -> (x .or. y?=w502:bool)
              }
              n273 = Path To String(path=w487) -> (string=w493:string[])
              n274 = Bundle By Name(cluster=T16 {"XYZ Positions"=[], "File Paths"=[]} ("Marked Positions"), "XYZ Positions"=w484, "File Paths"=w493) -> (w492:T16)
              n275 = Flatten To JSON(anything=w492) -> (JSON string=w491:string, 11:w489:errorcluster)  [unwired: 2 in]
              n276 = Write to Text File(file (use dialog)=w483, text=w491, error in=w489) -> (refnum out=w490:refnum<file>, error out=w488:errorcluster)  [unwired: 1 in, 1 out]
              n277 = Close File(refnum=w490, error in=w488) -> ()  [unwired: 2 out]
            }
            frame "Clear All" {
              n278 = Flatten To JSON(anything=T16 {"XYZ Positions"=[], "File Paths"=[]} ("Marked Positions")) -> (JSON string=w515:string, 11:w513:errorcluster)  [unwired: 2 in]
              n279 = Write to Text File(file (use dialog)=w510, text=w515, error in=w513) -> (refnum out=w514:refnum<file>, error out=w512:errorcluster)  [unwired: 1 in, 1 out]
              n280 = Close File(refnum=w514, error in=w512) -> ()  [unwired: 2 out]
              n281 = Initialize Array(path "", 0 ("dimension size")) -> (w518:path[])
            }
            frame "Abort" {
              n282 = property on="Marked Positions" class="MCListbox (strict)"() -> ("ItemNames"=w524:string[][], "Value"=w521:i32)  [unwired: 2 in, 2 out]
              n283 = Get Notifier Status(notifier=w533) -> (notifier out=w529:refnum<notifier>, current notification=w532:T1)  [unwired: 1 in, 3 out]
              n284 = Bundle By Name(cluster=w532, "Actions"=Orca_Flash_Capture_Actions."Abort", "Running?"=FALSE) -> (w528:T1)
              n285 = Replace Array Subset(array=w524, new element="Abort" ("new element/subarray"), index (row)=w521, index (col)=5 ("disabled index (col)")) -> (w525:string[][])
              n286 = property on="Marked Positions" class="MCListbox (strict)"("ItemNames"=w525) -> ()  [unwired: 2 in, 2 out]
              n287 = Send Notification(notification=w528, notifier=w529) -> (notifier out=w527:refnum<notifier>)  [unwired: 1 in, 1 out]
              n288 = for {
                N: 600 -> [_]
                tunnel: w527 -> [w541]
                stop <- w538 stop-if-true
                n289 = Get Notifier Status(notifier=w541) -> (# waiting=w540:i32)  [unwired: 1 in, 4 out]
                n290 = Wait (ms)(milliseconds to wait=u32 10) -> ()  [unwired: 1 out]
                n291 = Greater Than 0?(x=w540) -> (x > 0?=w538:bool)
              }
            }
            frame "Quit" {
              n292 = case shown="No Error" w545 {
                tunnel: w547 -> [w551 _]
                tunnel: w546 -> [w550 _]
                frame No Error {
                  n293 = Release Notifier(notifier=w551) -> ()  [unwired: 2 in, 3 out]
                  n294 = Release Notifier(notifier=w550) -> ()  [unwired: 2 in, 3 out]
                }
                frame Error {
                }
              }
              n295 = Release Notifier(notifier=w544) -> ()  [unwired: 2 in, 3 out]
            }
          }
        }
      }
      n296 = local write "Quit"(w106) -> ()
    }
    frame Error {
      w702 = "\r"
      n297 = Release Notifier(notifier=w704, error in (no error)=w703) -> (error out=w700:errorcluster)  [unwired: 1 in, 2 out]
      n298 = Unbundle By Name(w700) -> ("source"=w699:string)
      n299 = Concatenate Strings("Image Multiple Areas had a startup error.", w702, w702, w699) -> (w698:string)
      n300 = One Button Dialog(message=w698) -> ()  [unwired: 1 in, 1 out]
    }
  }
  n301 = control-ref of="This VI"() -> (w21:refnum<vi>)
  n302 = property class="VI"(reference=w21) -> (reference out=w30:refnum<vi>, "Panel"=w22:refnum<vi>)  [unwired: 1 in, 1 out]
  n303 = property class="Pnl"(reference=w22) -> ("Decos[]"=w20:refnum<vi>[], "Panes[]"=w26:refnum<vi>[])  [unwired: 1 in, 2 out]
  n304 = Array Size(array=w20) -> (size(s)=w18:i32)
  n305 = Decrement(x=w18) -> (x-1=w19:i32)
  n306 = Index Array(array=w26, index=0) -> (element=w25:refnum<vi>)
  n307 = Index Array(array=w20, index=w19) -> (element=w28:refnum<vi>)
  n308 = property class="VI"(reference=w30) -> (reference out=w32:refnum<vi>, "Front Panel.PanelBounds"=w33:T20)  [unwired: 1 in, 1 out]
  n309 = property class="Decor"(reference=w28) -> ("Bounds"=w31:T21)  [unwired: 1 in, 2 out]
  n310 = property class="Pane"(reference=w25, "Origin"=T6 {"Horizontal"=0, "Vertical"=0}, "HorizScrollbarVisibility"=w29, "VertScrollbarVisibility"=w29) -> ()  [unwired: 1 in, 2 out]
  n311 = Unbundle By Name(w31) -> ("Width"=w36:u32, "Height"=w39:u32)
  n312 = control-ref of="Quit"() -> (w23:refnum<vi>)
  n313 = To Word Integer(number=w36) -> (16bit integer=w38:i16)
  n314 = To Word Integer(number=w39) -> ()  [unwired: 1 out]
  n315 = property class="Bool (strict)"(reference=w23) -> ("Height"=w41:u32, "Top"=w42:i32)  [unwired: 1 in, 2 out]
  n316 = Unbundle By Name(w33) -> ("Left"=w35:i16, "Top"=w46:i16)
  n317 = To Word Integer(number=w41) -> (16bit integer=w44:i16)
  n318 = To Word Integer(number=w42) -> (16bit integer=w45:i16)
  n319 = Add(x=w35, y=w38) -> (x+y=w37:i16)
  n320 = Compound Arithmetic op=ADD(w46, w44, w45, i16 12 ("y")) -> (w40:i16)
  n321 = Bundle By Name(cluster=w33, "Right"=w37, "Bottom"=w40) -> (w34:T20)
  n322 = property class="VI"(reference=w32, "Front Panel.PanelBounds"=w34) -> ()  [unwired: 1 in, 2 out]
